vi "Pair Index.vi"(11 "Pair":u8[](array[numeric])) -> (3 "Index":i32)   [LabVIEW 2020]
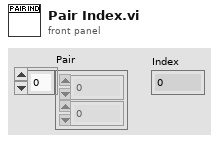
[diagram p1: front panel]
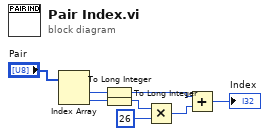
[diagram p0: block diagram]
diagram:
  n1 = Index Array(array="Pair") -> (element #1=w7:u8, element #2=w6:u8)  [unwired: 2 in]
  n2 = To Long Integer(number=w7) -> (32bit integer=w3:i32)
  n3 = To Long Integer(number=w6) -> (32bit integer=w5:i32)
  n4 = Multiply(x=w5, y=26) -> (x*y=w2:i32)
  n5 = Add(x=w3, y=w2) -> (x+y=→"Index":i32)
